vi "Read Frame.vi"(8 "error in (no error)":errorcluster, 9 "Timeout ms":i32, 11 "WebsocketStream in":refnum<class "WebsocketStream.lvclass">) -> (0 "error out":errorcluster, 1 "Remaining  Timeout":i32, 2 "Frame":T1, 3 "WebsocketStream out":refnum<class "WebsocketStream.lvclass">)   [LabVIEW 2020, in "Stream-Websocket.lvlib" / "WebsocketStream.lvclass"]
uses:
  WebsocketStream.lvclass
  WebsocketStream.lvclass/WebsocketStream.ctl
  OpCode.ctl
  Stream-Websocket.lvlib
  Message Frame.ctl
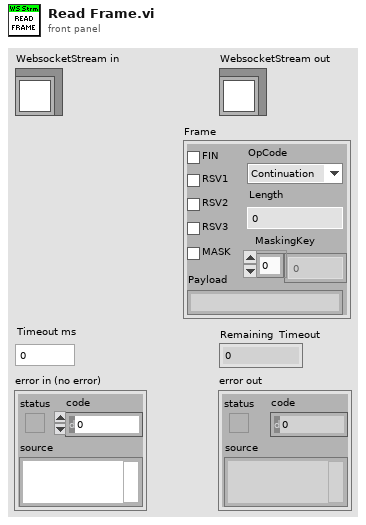
[diagram p1: front panel]
types:
  T1 = typedef "Stream-Websocket.lvlib/Message Frame.ctl" = cluster{"FIN":bool, "RSV1":bool, "RSV2":bool, "RSV3":bool, "MASK":bool, "OpCode":T2, "Length":u64, "MaskingKey":u8[], "Payload":string}
  T2 = typedef "Stream-Websocket.lvlib/OpCode.ctl" = enum8{"Continuation", "Text", "Binary", "Reserved3", "Reserved4", "Reserved5", "Reserved6", "Reserved7", "Close", "Ping", "Pong", "ReservedB", "ReservedC", "ReservedD", "ReservedE", "ReservedF"}
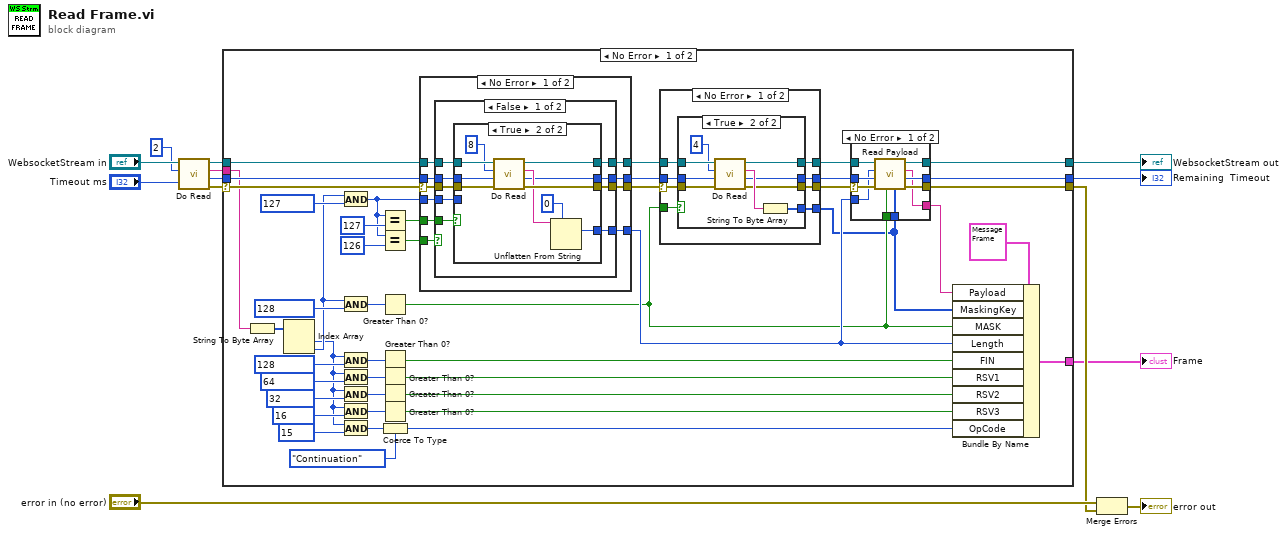
[diagram p0: block diagram]
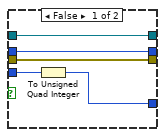
[diagram p5: hidden frame]
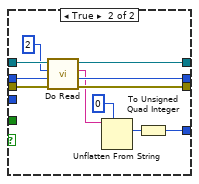
[diagram p6: hidden frame]
diagram:
  n1 = call "Do Read.vi"("Timeout ms"="Timeout ms", "Count"=2, "WebsocketStream in"="WebsocketStream in") -> ("error out"=w9:errorcluster, "Remaining  Timeout"=w8:i32, "Data"=w10:string, "WebsocketStream out"=w7:refnum<class "WebsocketStream.lvclass">)  [unwired: 5 in]
  n2 = case shown="No Error" w9 {
    selector: w9 -> [w58 w144]
    tunnel: w10 -> [w57 _]
    tunnel: w8 -> [w59 w145]
    tunnel: w7 -> [w28 w146]
    tunnel: [w20 w146] -> w6
    tunnel: [w19 w144] -> w3
    tunnel: [w18 w145] -> w5
    tunnel: [w24 _] -> w2
    frame No Error {
      n3 = String To Byte Array(string=w57) -> (unsigned byte array=w56:u8[])
      n4 = Index Array(array=w56) -> (element #1=w47:u8, element #2=w52:u8)  [unwired: 2 in]
      n5 = And(x=w52, y=u8 127) -> (x .and. y?=w29:u8)
      n6 = And(x=w52, y=u8 128) -> (x .and. y?=w42:u8)
      n7 = And(x=w47, y=u8 128) -> (x .and. y?=w43:u8)
      n8 = And(x=w47, y=u8 64) -> (x .and. y?=w44:u8)
      n9 = And(x=w47, y=u8 32) -> (x .and. y?=w45:u8)
      n10 = And(x=w47, y=u8 16) -> (x .and. y?=w46:u8)
      n11 = And(x=w47, y=u8 15) -> (x .and. y?=w36:u8)
      n12 = Equal?(x=w29, y=u8 127) -> (x = y?=w31:bool)
      n13 = Equal?(x=w29, y=u8 126) -> (x = y?=w30:bool)
      n14 = Greater Than 0?(x=w42) -> (x > 0?=w15:bool)
      n15 = Greater Than 0?(x=w43) -> (x > 0?=w40:bool)
      n16 = Greater Than 0?(x=w44) -> (x > 0?=w39:bool)
      n17 = Greater Than 0?(x=w45) -> (x > 0?=w38:bool)
      n18 = Greater Than 0?(x=w46) -> (x > 0?=w37:bool)
      n19 = Coerce To Type(0:w36, 1:OpCode."Continuation" ("OpCode")) -> (2:w35:T2)
      n20 = case shown="No Error" w58 {
        selector: w58 -> [w104 w141]
        tunnel: w59 -> [w105 w142]
        tunnel: w31 -> [w103 _]
        tunnel: w30 -> [w102 _]
        tunnel: w29 -> [w101 _]
        tunnel: w28 -> [w100 w143]
        tunnel: [w99 w141] -> w27
        tunnel: [w98 w142] -> w26
        tunnel: [w97 w143] -> w25
        tunnel: [w96 _] -> w16
        frame No Error {
          n21 = case shown="False" w102 {
            tunnel: w101 -> [w114 _]
            tunnel: w100 -> [w113 w140]
            tunnel: w105 -> [w112 w139]
            tunnel: w104 -> [w111 w138]
            tunnel: w103 -> [w110 _]
            tunnel: [w109 w131] -> w96
            tunnel: [w108 w134] -> w99
            tunnel: [w107 w135] -> w98
            tunnel: [w106 w136] -> w97
            frame False {
              n22 = case shown="True" w110 {
                tunnel: w114 -> [w119 _]
                tunnel: w113 -> [w117 w129]
                tunnel: w112 -> [w116 w128]
                tunnel: w111 -> [w115 w127]
                tunnel: [w118 w124] -> w109
                tunnel: [w115 w123] -> w108
                tunnel: [w116 w121] -> w107
                tunnel: [w117 w120] -> w106
                frame False {
                  n23 = To Unsigned Quad Integer(1:w119) -> (0:w118:u64)
                }
                frame True {
                  n24 = call "Do Read.vi"("error in (no error)"=w127, "Timeout ms"=w128, "Count"=8, "WebsocketStream in"=w129) -> ("error out"=w123:errorcluster, "Remaining  Timeout"=w121:i32, "Data"=w122:string, "WebsocketStream out"=w120:refnum<class "WebsocketStream.lvclass">)  [unwired: 4 in]
                  n25 = Unflatten From String(type=u64 0 ("Count"), binary string=w122) -> (value=w124:u64)  [unwired: 3 in, 2 out]
                }
              }
            }
            frame True {
              n26 = call "Do Read.vi"("error in (no error)"=w138, "Timeout ms"=w139, "Count"=2, "WebsocketStream in"=w140) -> ("error out"=w134:errorcluster, "Remaining  Timeout"=w135:i32, "Data"=w130:string, "WebsocketStream out"=w136:refnum<class "WebsocketStream.lvclass">)  [unwired: 4 in]
              n27 = Unflatten From String(type=u16 0 ("Count"), binary string=w130) -> (value=w132:u16)  [unwired: 3 in, 2 out]
              n28 = To Unsigned Quad Integer(1:w132) -> (0:w131:u64)
            }
          }
        }
        frame Error {
        }
      }
      n29 = case shown="No Error" w27 {
        selector: w27 -> [w80 w95]
        tunnel: w26 -> [w79 w94]
        tunnel: w25 -> [w78 w93]
        tunnel: w15 -> [w77 _]
        tunnel: [w76 _] -> w14
        tunnel: [w75 w93] -> w23
        tunnel: [w74 w95] -> w22
        tunnel: [w73 w94] -> w21
        frame No Error {
          n30 = case shown="True" w77 {
            tunnel: w80 -> [w81 w90]
            tunnel: w79 -> [w82 w91]
            tunnel: w78 -> [w83 w92]
            tunnel: [_ w87] -> w76
            tunnel: [w81 w86] -> w74
            tunnel: [w83 w85] -> w75
            tunnel: [w82 w84] -> w73
            frame False {
            }
            frame True {
              n31 = call "Do Read.vi"("error in (no error)"=w90, "Timeout ms"=w91, "Count"=4, "WebsocketStream in"=w92) -> ("error out"=w86:errorcluster, "Remaining  Timeout"=w84:i32, "Data"=w88:string, "WebsocketStream out"=w85:refnum<class "WebsocketStream.lvclass">)  [unwired: 4 in]
              n32 = String To Byte Array(string=w88) -> (unsigned byte array=w87:u8[])
            }
          }
        }
        frame Error {
        }
      }
      n33 = case shown="No Error" w22 {
        selector: w22 -> [w67 w71]
        tunnel: w23 -> [w69 w70]
        tunnel: w21 -> [w68 w72]
        tunnel: [w62 w70] -> w20
        tunnel: [w63 w71] -> w19
        tunnel: [w61 w72] -> w18
        tunnel: [w60 _] -> w17
        tunnel: w16 -> [w66 _]
        tunnel: w15 -> [w65 _]
        tunnel: w14 -> [w64 _]
        frame No Error {
          n34 = call "Read Payload.vi"("MaskingKey"=w64, "Mask"=w65, "error in (no error)"=w67, "Timeout ms"=w68, "Count"=w66, "WebsocketStream in"=w69) -> ("error out"=w63:errorcluster, "Remaining  Timeout"=w61:i32, "Data"=w60:string, "WebsocketStream out"=w62:refnum<class "WebsocketStream.lvclass">)  [unwired: 2 in]
        }
        frame Error {
        }
      }
      n35 = Bundle By Name(cluster=T1 {"FIN"=FALSE, "RSV1"=FALSE, "RSV2"=FALSE, "RSV3"=FALSE, "MASK"=FALSE, "OpCode"=enum."Continuation", "Length"=0, "MaskingKey"=[], "Payload"=""} ("Message Frame"), "Payload"=w17, "MaskingKey"=w14, "MASK"=w15, "Length"=w16, "FIN"=w40, "RSV1"=w39, "RSV2"=w38, "RSV3"=w37, "OpCode"=w35) -> (w24:T1)
    }
    frame Error {
    }
  }
  "WebsocketStream out" <- w6
  "Remaining  Timeout" <- w5
  "Frame" <- w2
  n36 = Merge Errors("error in (no error)", w3) -> (→"error out":errorcluster)
